vi "Initialize.vi"(8 "error in":errorcluster, 10 "parameters":variant, 11 "node in":refnum<class "ActiveFrontEndModule editor node.lvclass">) -> (0 "error out":errorcluster, 2 "summary":T2[](array[typedef]), 3 "data value reference":T1)   [LabVIEW 2017, in "ActiveFrontEndModule editor node.lvclass"]
doc: "Initializes the data of a node to its default state.\nThe object is not created inside of this VI, because it is created from a File depending on user selection."
uses:
  ActiveFrontEndModule editor node.lvclass
  C:/Program Files (x86)/National Instruments/LabVIEW 2017/vi.lib/NI/Configuration Framework/Node/NISE_CEF_Node.lvclass
  <vilib>/NI/Configuration Framework/Node/Summary.ctl
  <vilib>/NI/Configuration Framework/Node/NodeRef.ctl
  <vilib>/NI/Configuration Framework/Node/NISE_CEF_Node.lvclass
  module/configuration/ActiveFrontEndModule configuration.lvclass
  C:/Program Files (x86)/National Instruments/LabVIEW 2017/vi.lib/NI/Configuration Framework/serializable configuration/NISE_CEF_serializable configuration.lvclass
  <vilib>/NI/PowerElectronicsControl/ActiveFrontEnd/AFE/Parameters.ctl
  <vilib>/NI/PowerElectronicsControl/ActiveFrontEnd/AFE/Mode.ctl
  <vilib>/NI/PowerElectronicsControl/ActiveFrontEnd/AFE/PI_Settings.ctl
  <vilib>/rvi/Analysis/control/PID/Typedef/niFpgaPID_PIGains.ctl
  <vilib>/rvi/Analysis/control/PID/Typedef/niFpgaPID_OutputRange.ctl
  module/configuration/ActiveFrontEndModule configuration.lvclass/ActiveFrontEndModule configuration.ctl
  module/configuration/Write Parameters.vi
  module/configuration/Write ID_to_VD.vi
  module/configuration/Write IQ_to_VQ.vi
  module/configuration/Write VDCLinkToPower.vi
  <vilib>/NI/DCAF/Tag Editor Core/control module/editor node/control module editor.lvclass
  <vilib>/NI/Configuration Framework/serializable configuration/NISE_CEF_serializable configuration.lvclass
  <vilib>/NI/PowerElectronicsControl/ActiveFrontEnd/AFE/ActiveFrontEnd.lvlib
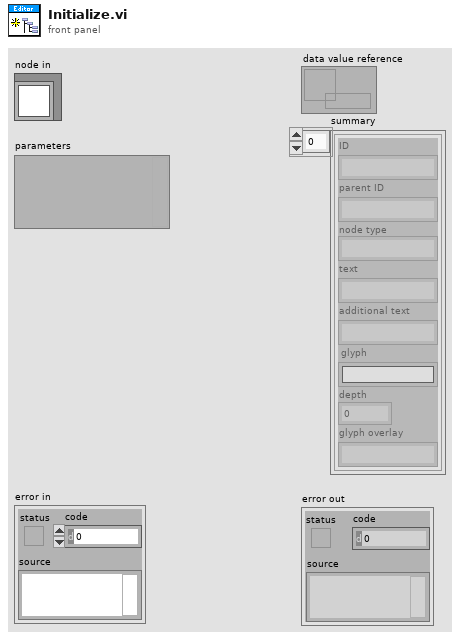
[diagram p1: front panel]
types:
  T1 = typedef "NISE_CEF_Node.lvclass/NodeRef.ctl" = refnum<data-value>
  T2 = typedef "NISE_CEF_Node.lvclass/Summary.ctl" = cluster{"ID":string, "parent ID":string, "node type":string, "text":string, "additional text":string, "glyph":string, "depth":i32, "glyph overlay":string}
  T3 = typedef "ActiveFrontEnd.lvlib/PI_Settings.ctl" = cluster{"gains":T4, "output range":T5, "PI_state":enum8{"idle", "normal", "manual", "perturbance"}, "reset":bool, "manual":sgl}
  T4 = typedef "niFpgaPID_PIGains.ctl" = cluster{"proportional gain":sgl, "integral gain":sgl}
  T5 = typedef "niFpgaPID_OutputRange.ctl" = cluster{"output high (Inf)":sgl, "output low (-Inf)":sgl}
  T6 = typedef "ActiveFrontEnd.lvlib/Parameters.ctl" = cluster{"VDCLink_setpt":sgl, "VDCLinkRampRate":sgl, "Q_setpt":sgl, "Pf_setpt":sgl, "Mode":T7, "perturbance_amp":sgl, "perturbance_freq":sgl, "dT":sgl}
  T7 = typedef "ActiveFrontEnd.lvlib/Mode.ctl" = enum16{"Q Control", "Pf Control"}
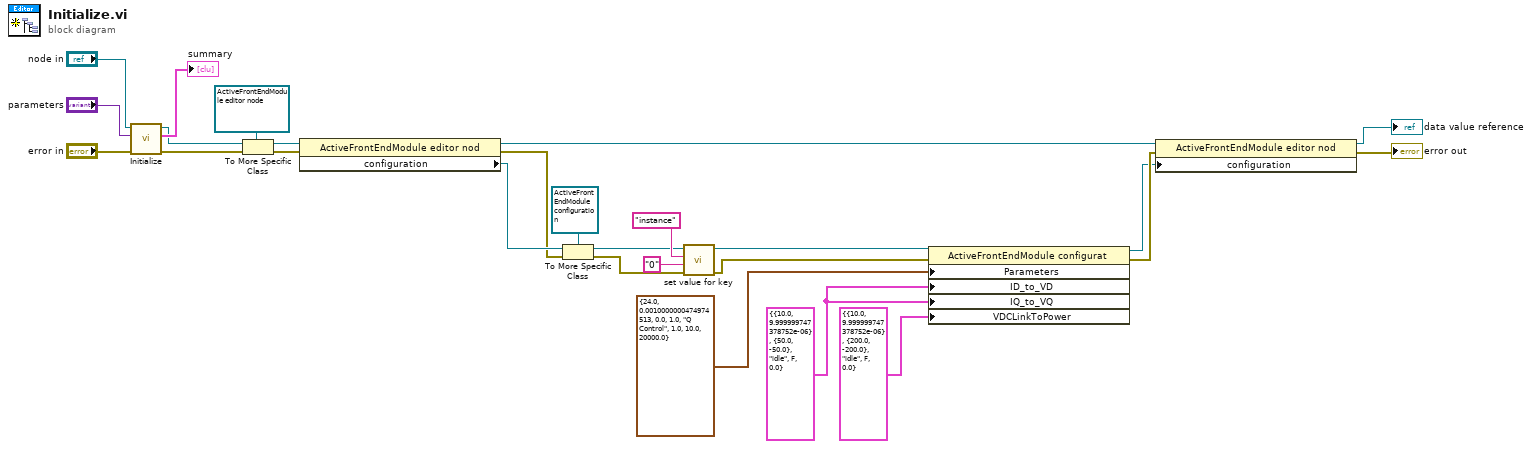
[diagram p0: block diagram]
diagram:
  w2 = T3 {"gains"={"proportional gain"=10.0, "integral gain"=1e-05}, "output range"={"output high (Inf)"=50.0, "output low (-Inf)"=-50.0}, "PI_state"=enum."idle", "reset"=FALSE, "manual"=0.0} ("ID_to_VD")
  n1 = call-parent "Initialize.vi"("error in"="error in", "parameters"="parameters", "node in"="node in") -> ("error out"=w22:errorcluster, "summary"=→"summary":T2[], "data value reference"=w21:T1)  [unwired: 6 in]
  n2 = To More Specific Class(target class=refnum<data-value> refnum ("data value reference"), reference=w21, error in=w22) -> (specific class reference=w19:refnum<data-value>, error out=w18:errorcluster)
  n3 = property class="ActiveFrontEndModule editor nod"(reference=w19, error in=w18) -> (reference out=w4:refnum<data-value>, error out=w11:errorcluster, "configuration"=w13:refnum<class "NISE_CEF_serializable configuration.lvclass">)
  n4 = To More Specific Class(target class=refnum<class "ActiveFrontEndModule configuration.lvclass"> refnum ("ActiveFrontEndModule configuration"), reference=w13, error in=w11) -> (specific class reference=w10:refnum<class "ActiveFrontEndModule configuration.lvclass">, error out=w9:errorcluster)
  n5 = call-dynamic "set value for key.vi"("error in"=w9, "value"="0", "key"="instance", "fixed channel configuration in"=w10) -> ("error out"=w7:errorcluster, "fixed channel configuration out"=w8:refnum<class "ActiveFrontEndModule configuration.lvclass">)  [unwired: 6 in]
  n6 = property class="ActiveFrontEndModule configurat"(reference=w8, error in=w7, "Parameters"=T6 {"VDCLink_setpt"=24.0, "VDCLinkRampRate"=0.001, "Q_setpt"=0.0, "Pf_setpt"=1.0, "Mode"=enum."Q Control", "perturbance_amp"=1.0, "perturbance_freq"=10.0, "dT"=20000.0}, "ID_to_VD"=w2, "IQ_to_VQ"=w2, "VDCLinkToPower"=T3 {"gains"={"proportional gain"=10.0, "integral gain"=1e-05}, "output range"={"output high (Inf)"=200.0, "output low (-Inf)"=-200.0}, "PI_state"=enum."idle", "reset"=FALSE, "manual"=0.0} ("ID_to_VD")) -> (reference out=w5:refnum<class "ActiveFrontEndModule configuration.lvclass">, error out=w6:errorcluster)
  n7 = property class="ActiveFrontEndModule editor nod"(reference=w4, error in=w6, "configuration"=w5) -> (reference out=→"data value reference":refnum<data-value>, error out=→"error out":errorcluster)
